vi "Write SentTimerToParent Msg.vi"(10 "Timer_Event.lvlib:SentTimerToParent Msg.lvclass":refnum<class "SentTimerToParent Msg.lvclass">, 11 "Timer_Event in":refnum<class "Timer_Event.lvclass">) -> (3 "Timer_Event out":refnum<class "Timer_Event.lvclass">)   [LabVIEW 2020, in "Timer_Event.lvlib" / "Timer_Event.lvclass"]
uses:
  Timer_Event.lvclass
  Timer_Event Messages/SentTimerToParent Msg/SentTimerToParent Msg.lvclass
  Timer_Event.lvclass/Timer_Event.ctl
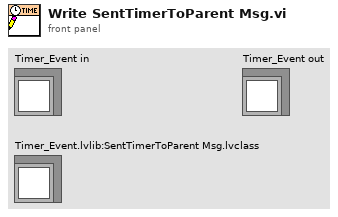
[diagram p1: front panel]
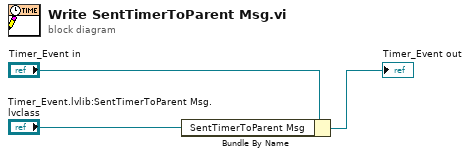
[diagram p0: block diagram]
diagram:
  n1 = Bundle By Name(cluster="Timer_Event in", "SentTimerToParent Msg"="Timer_Event.lvlib:SentTimerToParent Msg.lvclass") -> (→"Timer_Event out":refnum<class "Timer_Event.lvclass">)
